vi "Sensor-Resistance-Sampling_withg.vi"(1 "hold time (sec)":dbl=10.0 format="%#_13g", 2 "Gate step - extra milliseconds to wait":u32=20000, 3 "Current through sensor (A)":dbl format="%#_13g", 4 "Number of times measurement is done":i32=7, 6 "Number of heater steps":i32=7, 7 "Heater Step (V)":dbl=3.3) -> ()   [LabVIEW 2016]
uses:
  <vilib>/Utility/file.llb/Write To Spreadsheet File (DBL).vi
  <vilib>/Utility/file.llb/Read From Spreadsheet File (DBL).vi
  Driver/New driver/Agilent 415X Series.lvlib
panel:
  in  "Gate Step":dbl=-6.0
  in  "Gate Start":dbl format="%#_13g"
  in  "number of samples per heater step":i32=10
  out "error out":errorcluster
  out "Voltage across heater (VSU 1 and SMU4)":dbl[][](graph)
  out "Voltage measured between SMU1 (Common) and SMU2":dbl[](graph)
  out "SPA VISA resource name":refnum<visa-resource-name>
  in  "1. SPA VISA resource name":refnum<visa-resource-name>="GPIB0::14::INSTR"
  in  "error in (no error)":errorcluster
  # "2. Heater Parameters"
  # "3. Repeat Entire Cycle"
  # "4. Timings \n(Should be same as those when sampling Thermopower)"
  # "5. Other measurement parameters"
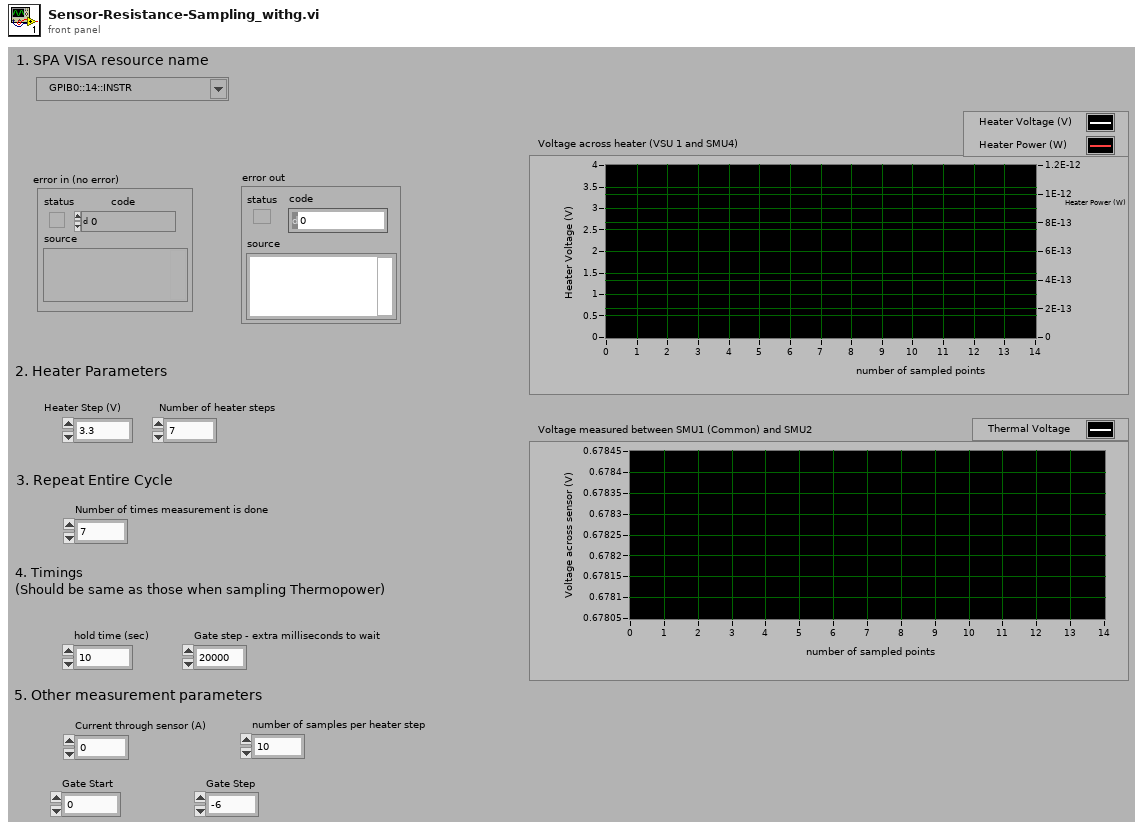
[diagram p1: front panel]
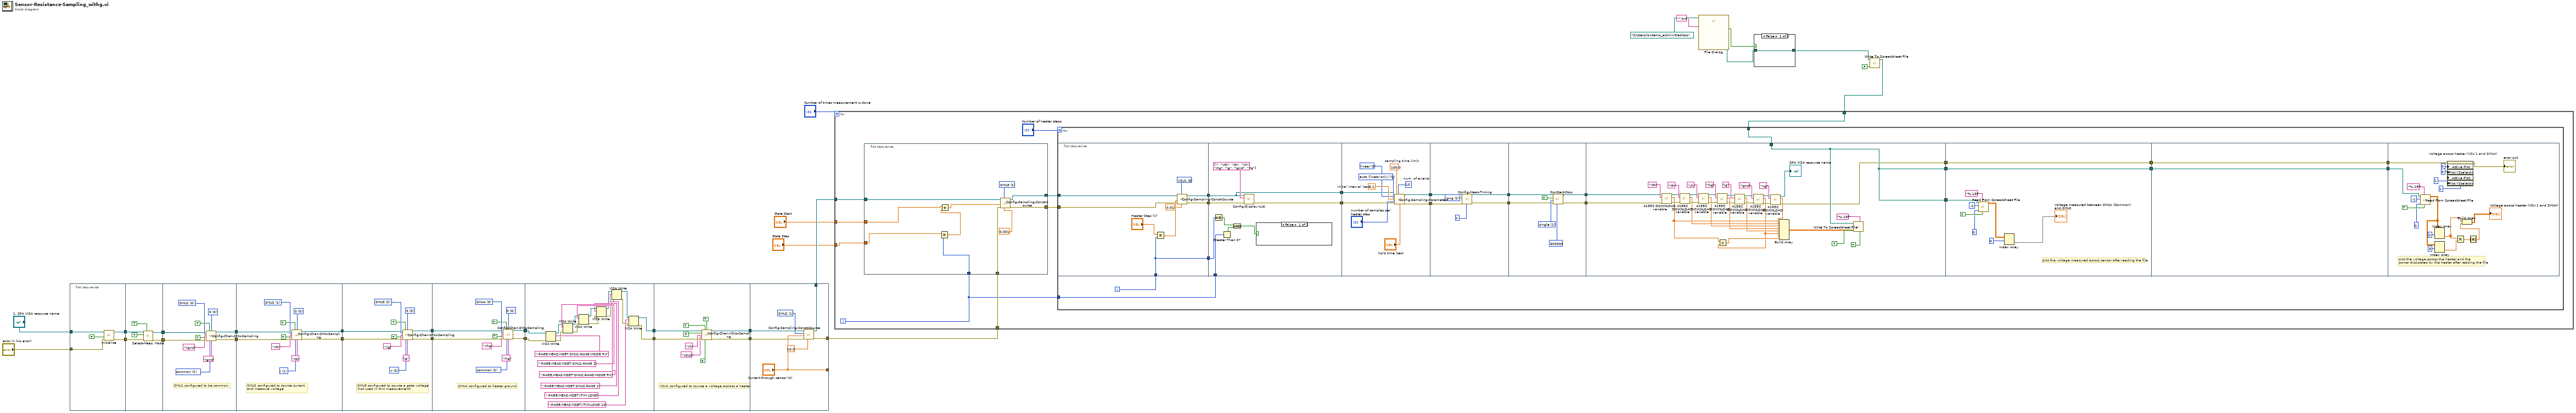
[diagram p0: block diagram]
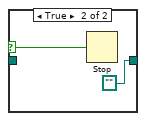
[diagram p2: hidden frame]
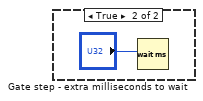
[diagram p3: hidden frame]
diagram:
  n1 = flat-sequence {
    tunnel: "error in (no error)" -> [w34]
    tunnel: "1. SPA VISA resource name" -> [w33]
    tunnel: [w32] -> w28
    tunnel: [w31] -> w27
    tunnel: w28 -> [w41]
    tunnel: w27 -> [w40]
    tunnel: [w37] -> w26
    tunnel: [w36] -> w25
    tunnel: w26 -> [w49]
    tunnel: w25 -> [w48]
    tunnel: [w47] -> w24
    tunnel: [w46] -> w23
    tunnel: w24 -> [w60]
    tunnel: w23 -> [w59]
    tunnel: [w58] -> w22
    tunnel: [w57] -> w21
    tunnel: w22 -> [w71]
    tunnel: w21 -> [w70]
    tunnel: [w69] -> w18
    tunnel: [w68] -> w17
    tunnel: w18 -> [w76]
    tunnel: [w77] -> w6
    tunnel: w17 -> [w75]
    tunnel: [w78] -> w4
    tunnel: w6 -> [w89]
    tunnel: [w86] -> w5
    tunnel: w4 -> [w88]
    tunnel: [w87] -> w3
    tunnel: w5 -> [w113]
    tunnel: w3 -> [w115]
    tunnel: [w114] -> w20
    tunnel: [w112] -> w19
    tunnel: w20 -> [w119]
    tunnel: w19 -> [w120]
    tunnel: [w118] -> w15
    tunnel: [w117] -> w14
    tunnel: ["Current through sensor (A)"] -> _
    frame #0 {
      n2 = call "Initialize.vi"("error in (no error)"=w34, "reset"=TRUE, "VISA resource name"=w33) -> ("error out"=w31:errorcluster, "VISA resource name out"=w32:refnum<visa-resource-name>)  [unwired: 2 in, 5 out]
    }
    frame #1 {
      n3 = call "Select-Meas. Mode.vi"("clear all channels"=TRUE, "error in (no error)"=w40, "measurement mode"=TRUE, "VISA resource name"=w41) -> ("error out"=w36:errorcluster, "VISA resource name out"=w37:refnum<visa-resource-name>)  [unwired: 1 in, 5 out]
    }
    frame #2 {
      w44 = 0 items=["0  ", "10K Ohms  ", "100K Ohms  ", "1M Ohms  "] ("series resistance *")
      w45 = 2 items=["V  ", "I  ", "  common  "] ("mode")
      w50 = 0 items=["SMU1  ", "SMU2  ", "SMU3  ", "SMU4  ", "SMU5  ", "SMU6  "] ("unit to configure")
      # "SMU1 configured to be common"
      n4 = call "Config-Chan-SMU-Sampling.vi"("VISA resource name in"=w49, "function"=TRUE, "series resistance *"=w44, "unit to configure"=w50, "V name (max 6 chars)"="Vgnd", "standby"=TRUE, "error in (no error)"=w48, "mode"=w45, "I name (max 6 chars)"="Ignd") -> ("VISA resource name out"=w47:refnum<visa-resource-name>, "error out"=w46:errorcluster)  [unwired: 5 out]
    }
    frame #3 {
      w54 = 0 items=["0  ", "10K Ohms  ", "100K Ohms  ", "1M Ohms  "] ("series resistance *")
      w56 = 1 items=["V  ", "I  ", "  common  "] ("mode")
      w61 = 1 items=["SMU1  ", "SMU2  ", "SMU3  ", "SMU4  ", "SMU5  ", "SMU6  "] ("unit to configure")
      # "SMU2 configured to source current \nand measure voltage"
      n5 = call "Config-Chan-SMU-Sampling.vi"("VISA resource name in"=w60, "function"=TRUE, "series resistance *"=w54, "unit to configure"=w61, "V name (max 6 chars)"="Vth", "standby"=TRUE, "error in (no error)"=w59, "mode"=w56, "I name (max 6 chars)"="Ith") -> ("VISA resource name out"=w58:refnum<visa-resource-name>, "error out"=w57:errorcluster)  [unwired: 5 out]
    }
    frame #4 {
      w65 = 0 items=["0  ", "10K Ohms  ", "100K Ohms  ", "1M Ohms  "] ("series resistance *")
      w67 = 0 items=["V  ", "I  ", "  common  "] ("mode")
      w72 = 2 items=["SMU1  ", "SMU2  ", "SMU3  ", "SMU4  ", "SMU5  ", "SMU6  "] ("unit to configure")
      # "SMU3 configured to source a gate voltage\n(not used in this measurement)"
      n6 = call "Config-Chan-SMU-Sampling.vi"("VISA resource name in"=w71, "function"=TRUE, "series resistance *"=w65, "unit to configure"=w72, "V name (max 6 chars)"="Vg", "standby"=TRUE, "error in (no error)"=w70, "mode"=w67, "I name (max 6 chars)"="Ig") -> ("VISA resource name out"=w69:refnum<visa-resource-name>, "error out"=w68:errorcluster)  [unwired: 5 out]
    }
    frame #5 {
      w80 = 0 items=["0  ", "10K Ohms  ", "100K Ohms  ", "1M Ohms  "] ("series resistance *")
      w82 = 2 items=["V  ", "I  ", "  common  "] ("mode")
      w83 = 3 items=["SMU1  ", "SMU2  ", "SMU3  ", "SMU4  ", "SMU5  ", "SMU6  "] ("unit to configure")
      # "SMU4 configured to heater ground"
      n7 = call "Config-Chan-SMU-Sampling.vi"("VISA resource name in"=w76, "function"=TRUE, "series resistance *"=w80, "unit to configure"=w83, "V name (max 6 chars)"="Vhg", "standby"=TRUE, "error in (no error)"=w75, "mode"=w82, "I name (max 6 chars)"="Ihg") -> ("VISA resource name out"=w77:refnum<visa-resource-name>, "error out"=w78:errorcluster)  [unwired: 5 out]
    }
    frame #6 {
      n8 = VISA Write(VISA resource name=w89, write buffer=":PAGE:MEAS:MSET:SMU1:RANG:MODE FIX", error in (no error)=w88) -> (VISA resource name out=w104:refnum<visa-resource-name>, error out=w101:errorcluster)  [unwired: 1 out]
      n9 = VISA Write(VISA resource name=w104, write buffer=":PAGE:MEAS:MSET:SMU1:RANG 2", error in (no error)=w101) -> (VISA resource name out=w103:refnum<visa-resource-name>, error out=w100:errorcluster)  [unwired: 1 out]
      n10 = VISA Write(VISA resource name=w103, write buffer=":PAGE:MEAS:MSET:SMU2:RANG:MODE FIX", error in (no error)=w100) -> (VISA resource name out=w102:refnum<visa-resource-name>, error out=w99:errorcluster)  [unwired: 1 out]
      n11 = VISA Write(VISA resource name=w102, write buffer=":PAGE:MEAS:MSET:SMU2:RANG 2", error in (no error)=w99) -> (VISA resource name out=w94:refnum<visa-resource-name>, error out=w93:errorcluster)  [unwired: 1 out]
      n12 = VISA Write(VISA resource name=w94, write buffer=":PAGE:MEAS:MSET:ITIM LONG", error in (no error)=w93) -> (VISA resource name out=w92:refnum<visa-resource-name>, error out=w91:errorcluster)  [unwired: 1 out]
      n13 = VISA Write(VISA resource name=w92, write buffer=":PAGE:MEAS:MSET:ITIM:LONG 10", error in (no error)=w91) -> (VISA resource name out=w86:refnum<visa-resource-name>, error out=w87:errorcluster)  [unwired: 1 out]
    }
    frame #7 {
      # "VSU1 configured to source a voltage accross a heater"
      n14 = call "Config-Chan-VSUs-Sampling.vi"("VISA session"=w113, "VSU1 function"=TRUE, "VSU2 standby"=TRUE, "VSU1 standby"=FALSE, "VSU1 V name \n(max 6 chars)"="Vh" ("V name (max 6 chars)"), "VSU2 V name \n(max 6 chars)"="VSU2" ("V name (max 6 chars)"), "error in (no error)"=w115, "VSU2 function"=FALSE) -> ("VISA resource name out"=w112:refnum<visa-resource-name>, "error out"=w114:errorcluster)  [unwired: 6 out]
    }
    frame #8 {
      w121 = u16 1 items=["SMU 1", "SMU2", "SMU3", "SMU4", "SMU5", "SMU6", "VSU1", "VSU2"] ("unit (SMU1:0)")
      n15 = call "Config-Sampling-Const-Source.vi"("compliance (SMUs only)"=10.0, "error in (no error)"=w119, "source (V or A)"="Current through sensor (A)", "unit (SMU1:0)"=w121, "VISA session"=w120) -> ("error out"=w117:errorcluster, "VISA resource name out"=w118:refnum<visa-resource-name>)  [unwired: 5 out]
    }
  }
  n16 = call "File Dialog"("start path"=path "C:/Users/lowtemp_admin/Desktop", "pattern (all files)"="*.txt") -> ("selected path"=w12:path, "cancelled"=w11:bool)  [unwired: 10 in, 2 out]
  n17 = case shown="False" w11 {
    selector: w11 -> [_ w125]
    tunnel: w12 -> [w123 _]
    tunnel: [w123 path ""] -> w8
    frame False {
    }
    frame True {
      n18 = Stop(stop? (T)=w125) -> ()
    }
  }
  n19 = call-poly <vilib>:"Write To Spreadsheet File.vi"("append to file? (new file:F)"=FALSE, "file path (dialog if empty)"=w8) -> ("new file path (Not A Path if cancelled)"=w7:path)  [unwired: 6 in]
  n20 = for {
    N: "Number of times measurement is done" -> [_]
    tunnel: w15 -> [w131]
    tunnel: w14 -> [w130]
    tunnel: w7 -> [w129]
    tunnel: "Gate Start" -> [w128]
    tunnel: "Gate Step" -> [w127]
    i -> [w126]
    n21 = flat-sequence {
      tunnel: w126 -> [w272]
      tunnel: [w277] -> w133
      tunnel: [w276] -> w132
      tunnel: w131 -> [w275]
      tunnel: w130 -> [w274]
      tunnel: w128 -> [w269]
      tunnel: w127 -> [w268]
      frame #0 {
        w278 = u16 2 items=["SMU 1", "SMU2", "SMU3", "SMU4", "SMU5", "SMU6", "VSU1", "VSU2"] ("unit (SMU1:0)")
        n22 = Multiply(x=w268, y=w272) -> (x*y=w271:dbl)
        n23 = Add(x=w269, y=w271) -> (x+y=w270:dbl)
        n24 = call "Config-Sampling-Const-Source.vi"("compliance (SMUs only)"=0.001, "error in (no error)"=w274, "source (V or A)"=w270, "unit (SMU1:0)"=w278, "VISA session"=w275) -> ("error out"=w276:errorcluster, "VISA resource name out"=w277:refnum<visa-resource-name>)  [unwired: 5 out]
      }
    }
    n25 = for {
      N: "Number of heater steps" -> [_]
      tunnel: w133 -> [w146]
      tunnel: w132 -> [w145]
      tunnel: w129 -> [w144]
      tunnel: w126 -> [w137]
      i -> [w147]
      n26 = flat-sequence {
        tunnel: [w165] -> w157
        tunnel: [w164] -> w156
        tunnel: w147 -> [w159]
        tunnel: w146 -> [w163]
        tunnel: w145 -> [w162]
        tunnel: [w159] -> w138
        tunnel: w157 -> [w174]
        tunnel: w156 -> [w172]
        tunnel: [w173] -> w155
        tunnel: [w172] -> w154
        tunnel: w138 -> [w168]
        tunnel: w137 -> [w167]
        tunnel: w155 -> [w180]
        tunnel: w154 -> [w179]
        tunnel: [w178] -> w153
        tunnel: [w177] -> w152
        tunnel: w153 -> [w191]
        tunnel: w152 -> [w190]
        tunnel: [w189] -> w151
        tunnel: [w188] -> w150
        tunnel: w151 -> [w197]
        tunnel: w150 -> [w196]
        tunnel: [w195] -> w149
        tunnel: [w194] -> w148
        tunnel: w149 -> [w218]
        tunnel: w148 -> [w217]
        tunnel: w144 -> [w219]
        tunnel: [w219] -> w143
        tunnel: [w219] -> w142
        tunnel: [w207] -> w140
        tunnel: w143 -> [w243]
        tunnel: [w238] -> w136
        tunnel: w142 -> [w238]
        tunnel: w140 -> [w239]
        tunnel: [w239] -> w135
        tunnel: [w248] -> w141
        tunnel: [w247] -> w139
        tunnel: w135 -> [w247]
        tunnel: w136 -> [w248]
        tunnel: w141 -> [w249]
        tunnel: w139 -> [w254]
        frame #0 {
          w166 = u16 6 items=["SMU 1", "SMU2", "SMU3", "SMU4", "SMU5", "SMU6", "VSU1", "VSU2"] ("unit (SMU1:0)")
          n27 = Multiply(x="Heater Step (V)", y=w159) -> (x*y=w160:dbl)
          n28 = call "Config-Sampling-Const-Source.vi"("compliance (SMUs only)"=0.01, "error in (no error)"=w162, "source (V or A)"=w160, "unit (SMU1:0)"=w166, "VISA session"=w163) -> ("error out"=w165:errorcluster, "VISA resource name out"=w164:refnum<visa-resource-name>)  [unwired: 5 out]
        }
        frame #1 {
          n29 = Equal To 0?(x=w168) -> (x = 0?=w169:bool)
          n30 = Greater Than 0?(x=w167) -> (x > 0?=w170:bool)
          n31 = And(x=w169, y=w170) -> (x .and. y?=w171:bool)
          n32 = call "Config-Display-List.vi"("error in (no error)"=w174, "list (max 8 elements)"=string[] ["", "Vth", "Ith", "Vh", "Ihg", "Ig", "Ignd", "Vg"], "VISA session"=w172) -> ("error out"=w173:errorcluster)  [unwired: 1 in, 7 out]
          n33 = case shown="False" w171 {
            frame False {
            }
            frame True {
              n34 = Wait (ms)(milliseconds to wait="Gate step - extra milliseconds to wait") -> ()  [unwired: 1 out]
            }
          }
        }
        frame #2 {
          w181 = 100.0  # sampling time limit
          w182 = 0 items=["linear", "log 10", "log 25", "log 50", "thinned out"] ("mode (linear: 0)")
          w183 = 0 items=["auto (linear only)", "no limit", "set limit "] ("sampling time\n(linear/thinned-out only)")
          w184 = 0.1  # initial interval (sec)
          w185 = 10  # num. of events
          n35 = call "Config-Sampling-Parameters.vi"("VISA session"=w179, "mode (linear: 0)"=w182, "initial interval (sec)"=w184, "sampling time\n(linear/thinned-out only)"=w183, "number of samples"="number of samples per heater step", "error in (no error)"=w180, "sampling time limit"=w181, "num. of events"=w185, "hold time (sec)"="hold time (sec)") -> ("VISA resource name out"=w177:refnum<visa-resource-name>, "error out"=w178:errorcluster)  [unwired: 7 in, 10 out]
        }
        frame #3 {
          w193 = 2 items=["short  ", "medium  ", "long  "] ("integration time")
          n36 = call "Config-Meas-Timing.vi"("# PLCs for long integration time"=1, "error in (no error)"=w191, "integration time"=w193, "VISA session"=w190) -> ("error out"=w189:errorcluster, "VISA resource name out"=w188:refnum<visa-resource-name>)  [unwired: 2 in, 4 out]
        }
        frame #4 {
          w199 = 1 items=["stop  ", "single  ", "single-append  ", "stress start  ", "continuous  ", "standby on  ", "standby off  ", "zero  "] ("function (stop:0)")
          n37 = call "Op-Start-Stop.vi"("time to wait (30000ms)"=600000, "error in (no error)"=w197, "function (stop:0)"=w199, "wait until finish"=TRUE, "VISA resource name"=w196) -> ("error out"=w195:errorcluster, "VISA resource name out"=w194:refnum<visa-resource-name>)  [unwired: 5 out]
        }
        frame #5 {
          n38 = call "4155C DOWNLOAD variable.vi"("error in (no error)"=w218, "Variable name"="Vth", "VISA resource name in"=w217) -> ("error out"=w227:errorcluster, "Output data"=w204:dbl[], "VISA Resource Name out"=w230:refnum<visa-resource-name>)  [unwired: 2 out]
          n39 = call "4155C DOWNLOAD variable.vi"("error in (no error)"=w227, "Variable name"="Ith", "VISA resource name in"=w230) -> ("error out"=w226:errorcluster, "Output data"=w224:dbl[], "VISA Resource Name out"=w229:refnum<visa-resource-name>)  [unwired: 2 out]
          n40 = call "4155C DOWNLOAD variable.vi"("error in (no error)"=w226, "Variable name"="Vh", "VISA resource name in"=w229) -> ("error out"=w225:errorcluster, "Output data"=w223:dbl[], "VISA Resource Name out"=w228:refnum<visa-resource-name>)  [unwired: 2 out]
          n41 = call "4155C DOWNLOAD variable.vi"("error in (no error)"=w225, "Variable name"="Ihg", "VISA resource name in"=w228) -> ("error out"=w212:errorcluster, "Output data"=w222:dbl[], "VISA Resource Name out"=w211:refnum<visa-resource-name>)  [unwired: 2 out]
          n42 = call "4155C DOWNLOAD variable.vi"("error in (no error)"=w212, "Variable name"="Ig", "VISA resource name in"=w211) -> ("error out"=w214:errorcluster, "Output data"=w202:dbl[], "VISA Resource Name out"=w215:refnum<visa-resource-name>)  [unwired: 2 out]
          n43 = call "4155C DOWNLOAD variable.vi"("error in (no error)"=w214, "Variable name"="Ignd", "VISA resource name in"=w215) -> ("error out"=w208:errorcluster, "Output data"=w201:dbl[], "VISA Resource Name out"=w209:refnum<visa-resource-name>)  [unwired: 2 out]
          n44 = Divide(x=w204, y=w201) -> (x/y=w203:dbl[])
          n45 = call "4155C DOWNLOAD variable.vi"("error in (no error)"=w208, "Variable name"="Vg", "VISA resource name in"=w209) -> ("error out"=w207:errorcluster, "Output data"=w205:dbl[], "VISA Resource Name out"=→"SPA VISA resource name":refnum<visa-resource-name>)  [unwired: 2 out]
          n46 = Build Array(w204, w224, w223, w222, w202, w201, w205, w203) -> (w221:dbl[][])
          n47 = call-poly <vilib>:"Write To Spreadsheet File.vi"("transpose? (no:F)"=TRUE, "format (%.3f)"="%.13f", "append to file? (new file:F)"=TRUE, "2D data"=w221, "file path (dialog if empty)"=w219) -> ()  [unwired: 1 in, 3 out]
        }
        frame #6 {
          # "plot the voltage measured across sensor after reading the file"
          n48 = call-poly <vilib>:"Read From Spreadsheet File.vi"("transpose (no:F)"=TRUE, "format (%.3f)"="%.13f", "max characters/row  (no limit:0)"=0, "number of rows (all:-1)"=-1, "file path (dialog if empty)"=w243) -> ("all rows"=w240:dbl[][])  [unwired: 6 out]
          n49 = Index Array(array=w240, index (row)=0) -> (element=→"Voltage measured between SMU1 (Common) and SMU2":dbl[])  [unwired: 1 in]
        }
        frame #7 {
        }
        frame #8 {
          # "plot the voltage across the heater and the \npower dissipated by the heater after reading the file"
          n50 = call-poly <vilib>:"Read From Spreadsheet File.vi"("transpose (no:F)"=TRUE, "format (%.3f)"="%.13f", "max characters/row  (no limit:0)"=0, "number of rows (all:-1)"=-1, "file path (dialog if empty)"=w249) -> ("all rows"=w262:dbl[][])  [unwired: 6 out]
          n51 = Index Array(array=w262, index (row)=2) -> (element=w256:dbl[])  [unwired: 1 in]
          n52 = Index Array(array=w262, index (row)=3) -> (element=w260:dbl[])  [unwired: 1 in]
          n53 = property on="Voltage across heater (VSU 1 and SMU4)" class="WFGraph (strict)"(error in=w254, "Active Plot"=u32 0, "Plot.YScaleIdx"=u32 0 ("Plot.Y Scale Index"), "Active Plot"=u32 1, "Plot.YScaleIdx"=u32 1 ("Plot.Y Scale Index")) -> (error out=→"error out":errorcluster)  [unwired: 1 in, 1 out]
          n54 = Multiply(x=w256, y=w260) -> (x*y=w259:dbl[])
          n55 = Absolute Value(x=w259) -> (abs(x)=w258:dbl[])
          n56 = Build Array(w256, w258) -> (→"Voltage across heater (VSU 1 and SMU4)":dbl[][])
        }
      }
    }
  }
